vi "题目1.vi"() -> ()   [LabVIEW 2017]
uses:
  <vilib>/measure/NI_MABase.lvlib
panel:
  in  "开关":bool
  out "波形图 2":waveform(dbl)(graph)
  out "波形图":waveform(dbl)(graph)
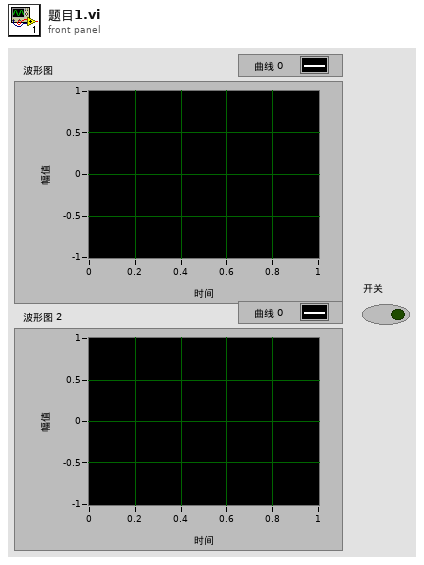
[diagram p1: front panel]
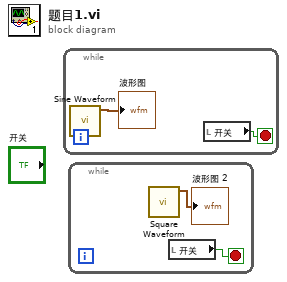
[diagram p0: block diagram]
diagram:
  n1 = while {
    stop <- w1 stop-if-true
    n2 = call <vilib>:"Sine Waveform.vi"() -> ("signal out"=→"波形图":waveform(dbl))  [unwired: 10 in, 1 out]
    n3 = local read "开关"() -> (w1:bool)
  }
  n4 = while {
    stop <- w3 stop-if-true
    n5 = call <vilib>:"Square Waveform.vi"() -> ("signal out"=→"波形图 2":waveform(dbl))  [unwired: 10 in, 1 out]
    n6 = local read "开关"() -> (w3:bool)
  }
